vi "Data Conversion - Byte Array to Signed 16 Bit Array.vi"(9 "Unsigned Byte Array":u8[](array[numeric]), 10 "Byte Order":T1(ring)) -> (2 "(Signed) 16 Bit Array":i16[](array[numeric]))   [LabVIEW 2017, in "Communications Library.lvlib"]
doc: "Converts a byte array into an array of 16 bit integers"
uses:
  Communications Library.lvlib
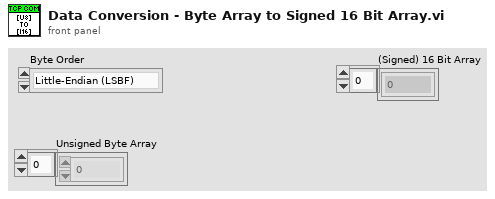
[diagram p1: front panel]
types:
  T1 = enum16{"Little-Endian (LSBF)", "Big-Endian (MSBF)"}
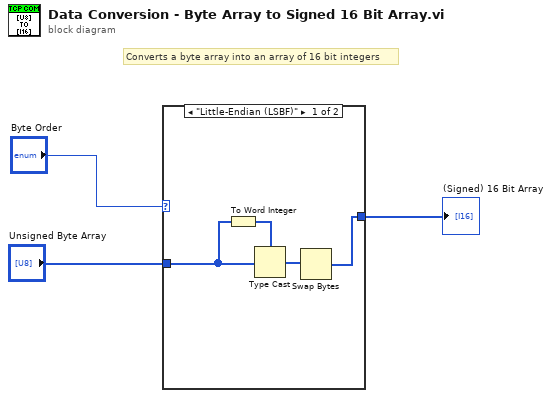
[diagram p0: block diagram]
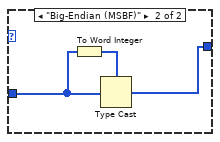
[diagram p2: hidden frame]
diagram:
  # "Converts a byte array into an array of 16 bit integers"
  n1 = case shown="\"Little-Endian (LSBF)\"" "Byte Order" {
    tunnel: "Unsigned Byte Array" -> [w7 w9]
    tunnel: [w4 w10] -> w1
    frame "Little-Endian (LSBF)" {
      n2 = To Word Integer(number=w7) -> (16bit integer=w6:i16[])
      n3 = Type Cast(type=w6, x=w7) -> (*(type *) &x=w5:i16[])
      n4 = Swap Bytes(anything=w5) -> (byte swapped=w4:i16[])
    }
    frame "Big-Endian (MSBF)" {
      n5 = To Word Integer(number=w9) -> (16bit integer=w8:i16[])
      n6 = Type Cast(type=w8, x=w9) -> (*(type *) &x=w10:i16[])
    }
  }
  "(Signed) 16 Bit Array" <- w1
